vi "FGGA TCP Packet_v3.3.vi"(0 "ID":string, 5 "Version":string, 7 "TCP Packet In":string, 9 "utc_time":u32, 12 "Data Array":string[](array[string])) -> (8 "TCP Binary Packet":string)   [LabVIEW 2014]
panel:
  out "array":string[](array[string])
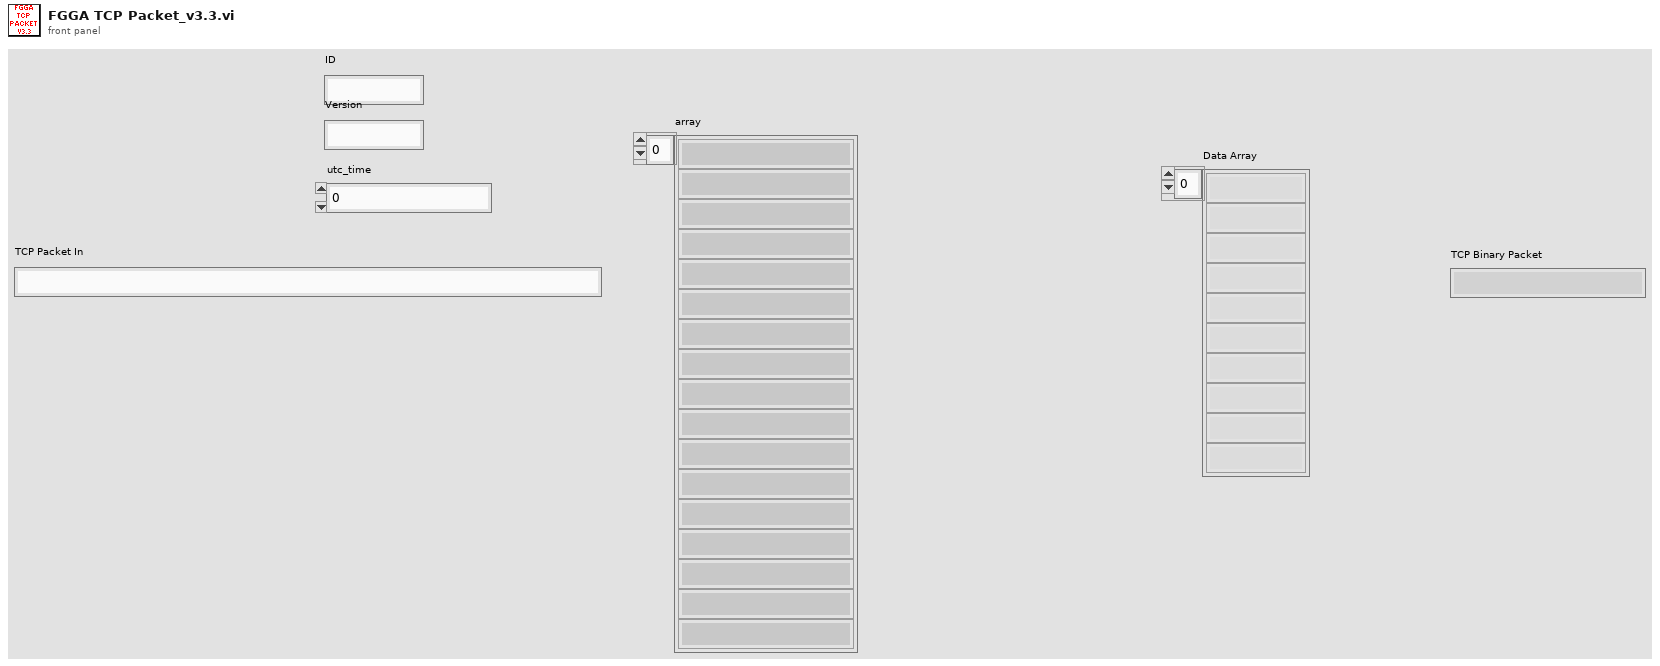
[diagram p1: front panel]
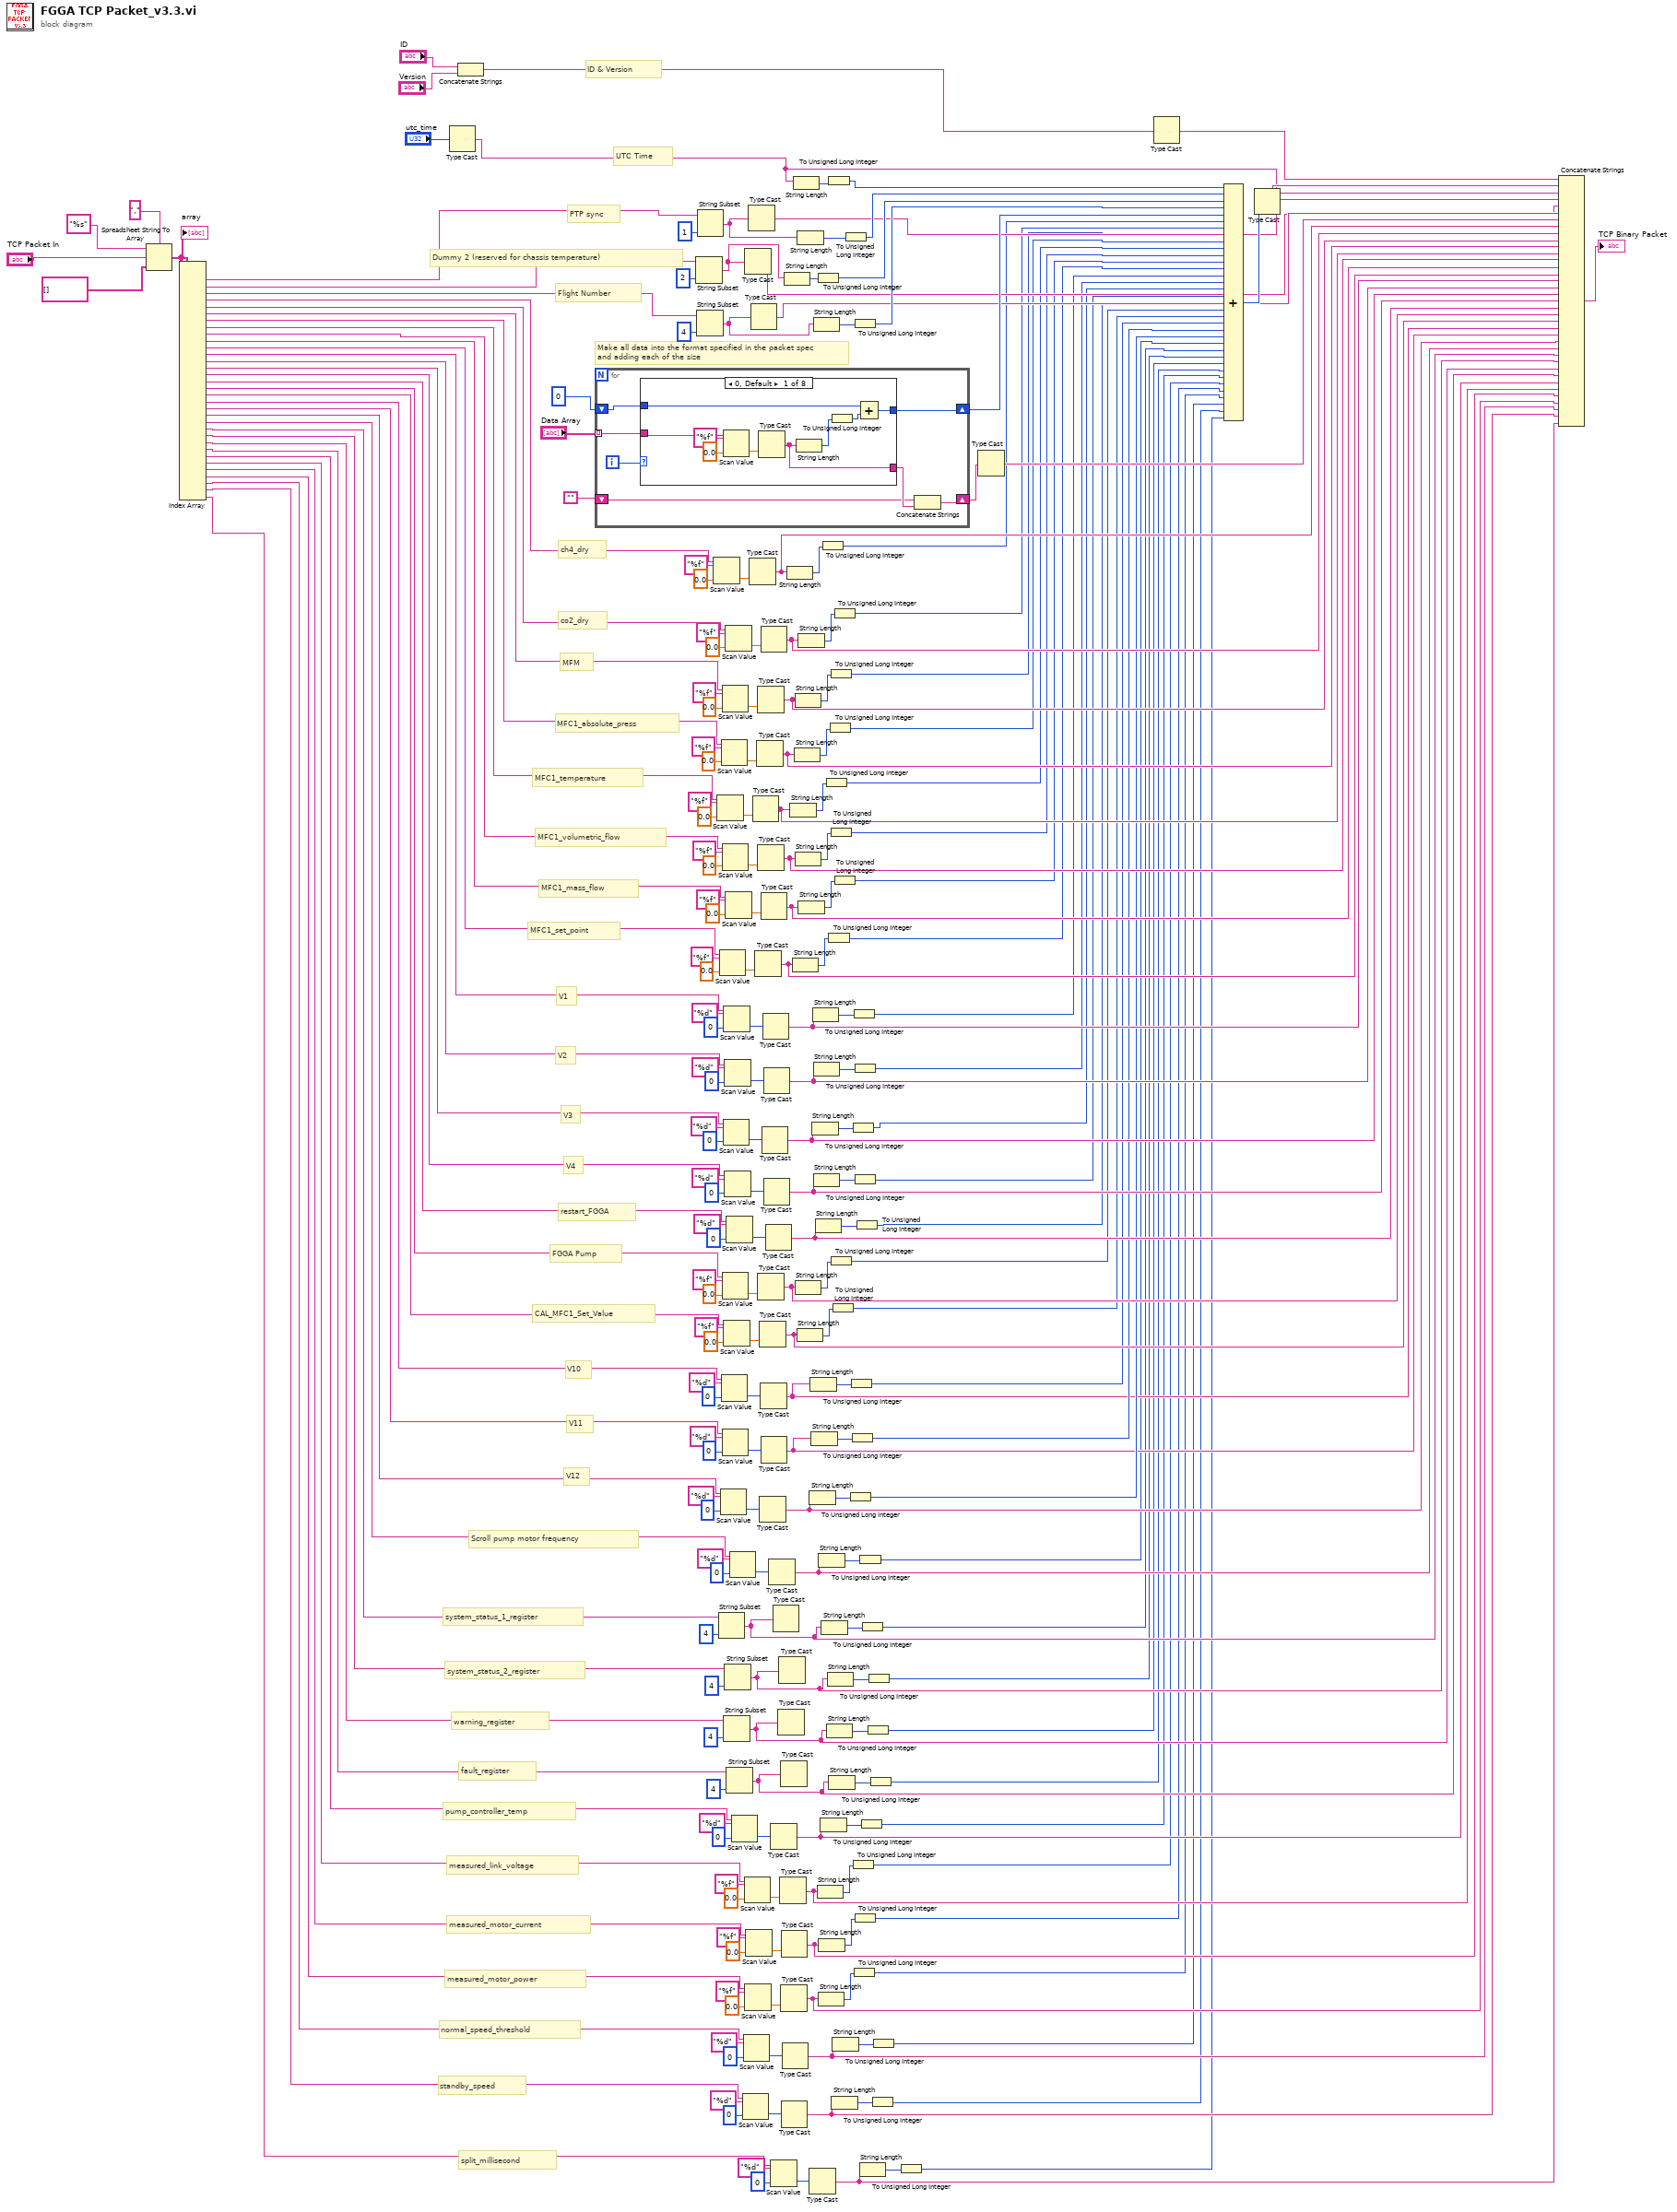
[diagram p0: block diagram]
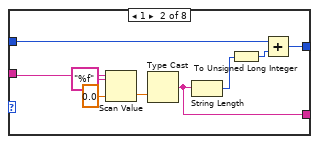
[diagram p2: hidden frame]
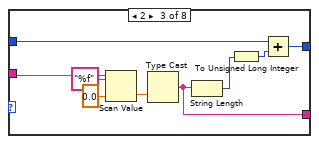
[diagram p3: hidden frame]
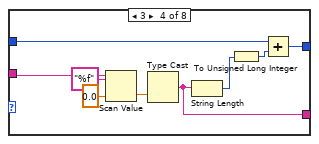
[diagram p4: hidden frame]
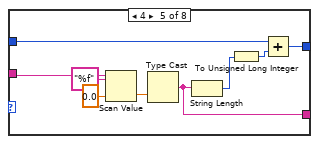
[diagram p5: hidden frame]
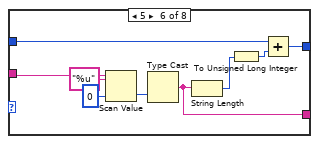
[diagram p6: hidden frame]
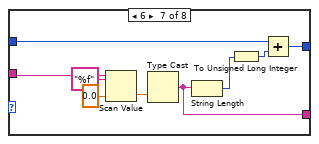
[diagram p7: hidden frame]
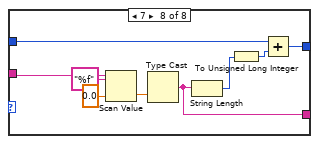
[diagram p8: hidden frame]
diagram:
  # "split_millisecond"
  # "standby_speed"
  # "normal_speed_threshold"
  # "measured_motor_power"
  # "measured_motor_current"
  # "measured_link_voltage"
  # "pump_controller_temp"
  # "fault_register"
  # "warning_register"
  # "system_status_2_register"
  # "system_status_1_register"
  # "Scroll pump motor frequency"
  # "V12"
  # "V11"
  # "V10"
  # "PTP sync"
  # "CAL_MFC1_Set_Value"
  # "FGGA Pump"
  # "restart_FGGA"
  # "V4"
  # "V3"
  # "V2"
  # "V1"
  # "MFC1_set_point"
  # "MFC1_mass_flow"
  # "MFC1_volumetric_flow"
  # "MFC1_temperature"
  # "MFC1_absolute_press"
  # "MFM"
  # "co2_dry"
  # "ch4_dry"
  # "Flight Number"
  # "Dummy 2 (reserved for chassis temperature)"
  # "UTC Time"
  # "ID & Version"
  # "Make all data into the format specified in the packet spec\nand adding each of the size"
  n1 = Spreadsheet String To Array(delimiter (Tab)=",", format string="%s", spreadsheet string="TCP Packet In", array type (2D Dbl)=string[] []) -> (array=w199:string[])
  "array" <- w199
  n2 = Index Array(array=w199) -> (element #1=w198:string, element #2=w197:string, element #3=w196:string, element #4=w195:string, element #5=w194:string, element #6=w169:string, element #7=w166:string, element #8=w163:string, element #9=w160:string, element #10=w157:string, element #11=w154:string, element #12=w147:string, element #13=w140:string, element #14=w117:string, element #15=w114:string, element #16=w111:string, element #17=w108:string, element #18=w105:string, element #19=w85:string, element #20=w84:string, element #21=w83:string, element #22=w40:string, element #23=w39:string, element #24=w38:string, element #25=w37:string, element #26=w36:string, element #27=w35:string, element #28=w34:string, element #29=w33:string, element #30=w32:string, element #31=w31:string, element #32=w30:string, element #33=w3:string)  [unwired: 33 in]
  n3 = Type Cast(x="utc_time") -> (*(type *) &x=w98:string)  [unwired: 1 in]
  n4 = Concatenate Strings("ID", "Version") -> (w100:string)
  n5 = for {
    tunnel: "Data Array" -> [w248] mode=indexing
    shift-right: [w246] -> w230
    shift-left: u32 0 -> [w247]
    shift-right: [w245] -> w219
    shift-left: "" -> [w243]
    i -> [w249]
    n6 = case shown="0, Default" w249 {
      tunnel: w248 -> [w256 w265 w274 w283 w292 w301 w310 w319]
      tunnel: w247 -> [w254 w263 w272 w281 w290 w299 w308 w317]
      tunnel: [w251 w260 w269 w278 w287 w296 w305 w314] -> w246
      tunnel: [w250 w259 w268 w277 w286 w295 w304 w313] -> w244
      frame 0, Default {
        n7 = Scan Value(string=w256, format string="%f", default (0 dbl)=sgl 0.0 ("default (0 I32)")) -> (value=w258:sgl)  [unwired: 1 out]
        n8 = Type Cast(x=w258) -> (*(type *) &x=w250:string)  [unwired: 1 in]
        n9 = String Length(string=w250) -> (length=w253:i32)
        n10 = To Unsigned Long Integer(number=w253) -> (unsigned 32bit integer=w252:u32)
        n11 = Add(x=w254, y=w252) -> (x+y=w251:u32)
      }
      frame 1 {
        n12 = Scan Value(string=w265, format string="%f", default (0 dbl)=sgl 0.0 ("default (0 I32)")) -> (value=w267:sgl)  [unwired: 1 out]
        n13 = Type Cast(x=w267) -> (*(type *) &x=w259:string)  [unwired: 1 in]
        n14 = String Length(string=w259) -> (length=w262:i32)
        n15 = To Unsigned Long Integer(number=w262) -> (unsigned 32bit integer=w261:u32)
        n16 = Add(x=w263, y=w261) -> (x+y=w260:u32)
      }
      frame 2 {
        n17 = Scan Value(string=w274, format string="%f", default (0 dbl)=sgl 0.0 ("default (0 I32)")) -> (value=w276:sgl)  [unwired: 1 out]
        n18 = Type Cast(x=w276) -> (*(type *) &x=w268:string)  [unwired: 1 in]
        n19 = String Length(string=w268) -> (length=w271:i32)
        n20 = To Unsigned Long Integer(number=w271) -> (unsigned 32bit integer=w270:u32)
        n21 = Add(x=w272, y=w270) -> (x+y=w269:u32)
      }
      frame 3 {
        n22 = Scan Value(string=w283, format string="%f", default (0 dbl)=sgl 0.0 ("default (0 I32)")) -> (value=w285:sgl)  [unwired: 1 out]
        n23 = Type Cast(x=w285) -> (*(type *) &x=w277:string)  [unwired: 1 in]
        n24 = String Length(string=w277) -> (length=w280:i32)
        n25 = To Unsigned Long Integer(number=w280) -> (unsigned 32bit integer=w279:u32)
        n26 = Add(x=w281, y=w279) -> (x+y=w278:u32)
      }
      frame 4 {
        n27 = Scan Value(string=w292, format string="%f", default (0 dbl)=sgl 0.0 ("default (0 I32)")) -> (value=w294:sgl)  [unwired: 1 out]
        n28 = Type Cast(x=w294) -> (*(type *) &x=w286:string)  [unwired: 1 in]
        n29 = String Length(string=w286) -> (length=w289:i32)
        n30 = To Unsigned Long Integer(number=w289) -> (unsigned 32bit integer=w288:u32)
        n31 = Add(x=w290, y=w288) -> (x+y=w287:u32)
      }
      frame 5 {
        n32 = Scan Value(string=w301, format string="%u", default (0 dbl)=u16 0 ("default (0 I32)")) -> (value=w303:u16)  [unwired: 1 out]
        n33 = Type Cast(x=w303) -> (*(type *) &x=w295:string)  [unwired: 1 in]
        n34 = String Length(string=w295) -> (length=w298:i32)
        n35 = To Unsigned Long Integer(number=w298) -> (unsigned 32bit integer=w297:u32)
        n36 = Add(x=w299, y=w297) -> (x+y=w296:u32)
      }
      frame 6 {
        n37 = Scan Value(string=w310, format string="%f", default (0 dbl)=sgl 0.0 ("default (0 I32)")) -> (value=w312:sgl)  [unwired: 1 out]
        n38 = Type Cast(x=w312) -> (*(type *) &x=w304:string)  [unwired: 1 in]
        n39 = String Length(string=w304) -> (length=w307:i32)
        n40 = To Unsigned Long Integer(number=w307) -> (unsigned 32bit integer=w306:u32)
        n41 = Add(x=w308, y=w306) -> (x+y=w305:u32)
      }
      frame 7 {
        n42 = Scan Value(string=w319, format string="%f", default (0 dbl)=sgl 0.0 ("default (0 I32)")) -> (value=w321:sgl)  [unwired: 1 out]
        n43 = Type Cast(x=w321) -> (*(type *) &x=w313:string)  [unwired: 1 in]
        n44 = String Length(string=w313) -> (length=w316:i32)
        n45 = To Unsigned Long Integer(number=w316) -> (unsigned 32bit integer=w315:u32)
        n46 = Add(x=w317, y=w315) -> (x+y=w314:u32)
      }
    }
    n47 = Concatenate Strings(w243, w244) -> (w245:string)
  }
  n48 = String Subset(string=w197, length (rest)=2 ("length (rest)")) -> (substring=w217:string)  [unwired: 1 in]
  n49 = String Subset(string=w196, length (rest)=4 ("length (rest)")) -> (substring=w223:string)  [unwired: 1 in]
  n50 = String Subset(string=w198, length (rest)=1 ("length (rest)")) -> (substring=w226:string)  [unwired: 1 in]
  n51 = Scan Value(string=w195, format string="%f", default (0 dbl)=sgl 0.0 ("default (0 I32)")) -> (value=w215:sgl)  [unwired: 1 out]
  n52 = Scan Value(string=w163, format string="%f", default (0 dbl)=sgl 0.0 ("default (0 I32)")) -> (value=w185:sgl)  [unwired: 1 out]
  n53 = String Subset(string=w39, length (rest)=4 ("length (rest)")) -> (substring=w26:string)  [unwired: 1 in]
  n54 = Scan Value(string=w154, format string="%f", default (0 dbl)=sgl 0.0 ("default (0 I32)")) -> (value=w173:sgl)  [unwired: 1 out]
  n55 = Scan Value(string=w83, format string="%d", default (0 dbl)=u16 0 ("default (0 I32)")) -> (value=w86:u16)  [unwired: 1 out]
  n56 = Scan Value(string=w166, format string="%f", default (0 dbl)=sgl 0.0 ("default (0 I32)")) -> (value=w189:sgl)  [unwired: 1 out]
  n57 = Scan Value(string=w85, format string="%d", default (0 dbl)=u16 0 ("default (0 I32)")) -> (value=w94:u16)  [unwired: 1 out]
  n58 = Scan Value(string=w169, format string="%f", default (0 dbl)=sgl 0.0 ("default (0 I32)")) -> (value=w193:sgl)  [unwired: 1 out]
  n59 = Scan Value(string=w160, format string="%f", default (0 dbl)=sgl 0.0 ("default (0 I32)")) -> (value=w181:sgl)  [unwired: 1 out]
  n60 = Scan Value(string=w108, format string="%f", default (0 dbl)=sgl 0.0 ("default (0 I32)")) -> (value=w125:sgl)  [unwired: 1 out]
  n61 = Scan Value(string=w84, format string="%d", default (0 dbl)=u16 0 ("default (0 I32)")) -> (value=w90:u16)  [unwired: 1 out]
  n62 = Scan Value(string=w117, format string="%d", default (0 dbl)=u16 0 ("default (0 I32)")) -> (value=w134:u16)  [unwired: 1 out]
  n63 = Scan Value(string=w147, format string="%d", default (0 dbl)=u16 0 ("default (0 I32)")) -> (value=w148:u16)  [unwired: 1 out]
  n64 = Scan Value(string=w105, format string="%f", default (0 dbl)=sgl 0.0 ("default (0 I32)")) -> (value=w121:sgl)  [unwired: 1 out]
  n65 = String Subset(string=w37, length (rest)=4 ("length (rest)")) -> (substring=w22:string)  [unwired: 1 in]
  n66 = Scan Value(string=w140, format string="%d", default (0 dbl)=u16 0 ("default (0 I32)")) -> (value=w141:u16)  [unwired: 1 out]
  n67 = Scan Value(string=w114, format string="%d", default (0 dbl)=u16 0 ("default (0 I32)")) -> (value=w130:u16)  [unwired: 1 out]
  n68 = String Subset(string=w38, length (rest)=4 ("length (rest)")) -> (substring=w24:string)  [unwired: 1 in]
  n69 = Scan Value(string=w194, format string="%f", default (0 dbl)=sgl 0.0 ("default (0 I32)")) -> (value=w209:sgl)  [unwired: 1 out]
  n70 = Scan Value(string=w157, format string="%f", default (0 dbl)=sgl 0.0 ("default (0 I32)")) -> (value=w177:sgl)  [unwired: 1 out]
  n71 = Scan Value(string=w111, format string="%d", default (0 dbl)=u16 0 ("default (0 I32)")) -> (value=w126:u16)  [unwired: 1 out]
  n72 = String Subset(string=w36, length (rest)=4 ("length (rest)")) -> (substring=w20:string)  [unwired: 1 in]
  n73 = Scan Value(string=w40, format string="%d", default (0 dbl)=u16 0 ("default (0 I32)")) -> (value=w73:u16)  [unwired: 1 out]
  n74 = Scan Value(string=w35, format string="%d", default (0 dbl)=u16 0 ("default (0 I32)")) -> (value=w61:u16)  [unwired: 1 out]
  n75 = Scan Value(string=w30, format string="%d", default (0 dbl)=u16 0 ("default (0 I32)")) -> (value=w41:u16)  [unwired: 1 out]
  n76 = Scan Value(string=w31, format string="%d", default (0 dbl)=u16 0 ("default (0 I32)")) -> (value=w45:u16)  [unwired: 1 out]
  n77 = Scan Value(string=w34, format string="%f", default (0 dbl)=sgl 0.0 ("default (0 I32)")) -> (value=w60:sgl)  [unwired: 1 out]
  n78 = Type Cast(x=w217) -> (*(type *) &x=w216:string)  [unwired: 1 in]
  n79 = Scan Value(string=w32, format string="%f", default (0 dbl)=sgl 0.0 ("default (0 I32)")) -> (value=w52:sgl)  [unwired: 1 out]
  n80 = Scan Value(string=w33, format string="%f", default (0 dbl)=sgl 0.0 ("default (0 I32)")) -> (value=w56:sgl)  [unwired: 1 out]
  n81 = Type Cast(x=w226) -> (*(type *) &x=w225:string)  [unwired: 1 in]
  n82 = Type Cast(x=w215) -> (*(type *) &x=w211:string)  [unwired: 1 in]
  n83 = Type Cast(x=w223) -> (*(type *) &x=w224:string)  [unwired: 1 in]
  n84 = Type Cast(x=w185) -> (*(type *) &x=w161:string)  [unwired: 1 in]
  n85 = Type Cast(x=w173) -> (*(type *) &x=w152:string)  [unwired: 1 in]
  n86 = Type Cast(x=w189) -> (*(type *) &x=w164:string)  [unwired: 1 in]
  n87 = Type Cast(x=w193) -> (*(type *) &x=w167:string)  [unwired: 1 in]
  n88 = Type Cast(x=w181) -> (*(type *) &x=w158:string)  [unwired: 1 in]
  n89 = Type Cast(x=w125) -> (*(type *) &x=w106:string)  [unwired: 1 in]
  n90 = Type Cast(x=w121) -> (*(type *) &x=w103:string)  [unwired: 1 in]
  n91 = Type Cast(x=w86) -> (*(type *) &x=w77:string)  [unwired: 1 in]
  n92 = Type Cast(x=w94) -> (*(type *) &x=w79:string)  [unwired: 1 in]
  n93 = Type Cast(x=w209) -> (*(type *) &x=w204:string)  [unwired: 1 in]
  n94 = Type Cast(x=w177) -> (*(type *) &x=w155:string)  [unwired: 1 in]
  n95 = Type Cast(x=w90) -> (*(type *) &x=w78:string)  [unwired: 1 in]
  n96 = Type Cast(x=w134) -> (*(type *) &x=w115:string)  [unwired: 1 in]
  n97 = Type Cast(x=w148) -> (*(type *) &x=w145:string)  [unwired: 1 in]
  n98 = Type Cast(x=w141) -> (*(type *) &x=w138:string)  [unwired: 1 in]
  n99 = Type Cast(x=w130) -> (*(type *) &x=w112:string)  [unwired: 1 in]
  n100 = Type Cast(x=w126) -> (*(type *) &x=w109:string)  [unwired: 1 in]
  n101 = Type Cast(x=w73) -> (*(type *) &x=w28:string)  [unwired: 1 in]
  n102 = Type Cast(x=w61) -> (*(type *) &x=w18:string)  [unwired: 1 in]
  n103 = Scan Value(string=w3, format string="%d", default (0 dbl)=u16 0 ("default (0 I32)")) -> (value=w4:u16)  [unwired: 1 out]
  n104 = Type Cast(x=w26) -> ()  [unwired: 1 in, 1 out]
  n105 = Type Cast(x=w22) -> ()  [unwired: 1 in, 1 out]
  n106 = Type Cast(x=w24) -> ()  [unwired: 1 in, 1 out]
  n107 = Type Cast(x=w60) -> (*(type *) &x=w16:string)  [unwired: 1 in]
  n108 = Type Cast(x=w20) -> ()  [unwired: 1 in, 1 out]
  n109 = Type Cast(x=w52) -> (*(type *) &x=w12:string)  [unwired: 1 in]
  n110 = Type Cast(x=w56) -> (*(type *) &x=w14:string)  [unwired: 1 in]
  n111 = Type Cast(x=w41) -> (*(type *) &x=w8:string)  [unwired: 1 in]
  n112 = Type Cast(x=w45) -> (*(type *) &x=w10:string)  [unwired: 1 in]
  n113 = String Length(string=w217) -> (length=w237:i32)
  n114 = String Length(string=w211) -> (length=w212:i32)
  n115 = String Length(string=w161) -> (length=w182:i32)
  n116 = String Length(string=w152) -> (length=w170:i32)
  n117 = String Length(string=w98) -> (length=w242:i32)
  n118 = String Length(string=w164) -> (length=w186:i32)
  n119 = String Length(string=w167) -> (length=w190:i32)
  n120 = String Length(string=w158) -> (length=w178:i32)
  n121 = String Length(string=w106) -> (length=w122:i32)
  n122 = String Length(string=w103) -> (length=w118:i32)
  n123 = String Length(string=w226) -> (length=w239:i32)
  n124 = String Length(string=w204) -> (length=w206:i32)
  n125 = String Length(string=w155) -> (length=w174:i32)
  n126 = String Length(string=w77) -> (length=w89:i32)
  n127 = Type Cast(x=w4) -> (*(type *) &x=w1:string)  [unwired: 1 in]
  n128 = String Length(string=w79) -> (length=w97:i32)
  n129 = String Length(string=w78) -> (length=w93:i32)
  n130 = String Length(string=w115) -> (length=w137:i32)
  n131 = String Length(string=w145) -> (length=w151:i32)
  n132 = String Length(string=w223) -> (length=w234:i32)
  n133 = String Length(string=w138) -> (length=w144:i32)
  n134 = String Length(string=w112) -> (length=w133:i32)
  n135 = To Unsigned Long Integer(number=w237) -> (unsigned 32bit integer=w236:u32)
  n136 = String Length(string=w109) -> (length=w129:i32)
  n137 = String Length(string=w16) -> (length=w57:i32)
  n138 = String Length(string=w12) -> (length=w49:i32)
  n139 = String Length(string=w28) -> (length=w76:i32)
  n140 = String Length(string=w14) -> (length=w53:i32)
  n141 = To Unsigned Long Integer(number=w212) -> (unsigned 32bit integer=w210:u32)
  n142 = String Length(string=w18) -> (length=w64:i32)
  n143 = String Length(string=w26) -> (length=w71:i32)
  n144 = To Unsigned Long Integer(number=w182) -> (unsigned 32bit integer=w162:u32)
  n145 = To Unsigned Long Integer(number=w242) -> (unsigned 32bit integer=w241:u32)
  n146 = To Unsigned Long Integer(number=w170) -> (unsigned 32bit integer=w153:u32)
  n147 = String Length(string=w22) -> (length=w67:i32)
  n148 = To Unsigned Long Integer(number=w186) -> (unsigned 32bit integer=w165:u32)
  n149 = String Length(string=w24) -> (length=w69:i32)
  n150 = To Unsigned Long Integer(number=w190) -> (unsigned 32bit integer=w168:u32)
  n151 = To Unsigned Long Integer(number=w178) -> (unsigned 32bit integer=w159:u32)
  n152 = To Unsigned Long Integer(number=w122) -> (unsigned 32bit integer=w107:u32)
  n153 = String Length(string=w20) -> (length=w65:i32)
  n154 = To Unsigned Long Integer(number=w118) -> (unsigned 32bit integer=w104:u32)
  n155 = To Unsigned Long Integer(number=w206) -> (unsigned 32bit integer=w205:u32)
  n156 = To Unsigned Long Integer(number=w174) -> (unsigned 32bit integer=w156:u32)
  n157 = String Length(string=w8) -> (length=w44:i32)
  n158 = String Length(string=w10) -> (length=w48:i32)
  n159 = To Unsigned Long Integer(number=w239) -> (unsigned 32bit integer=w238:u32)
  n160 = To Unsigned Long Integer(number=w89) -> (unsigned 32bit integer=w80:u32)
  n161 = To Unsigned Long Integer(number=w97) -> (unsigned 32bit integer=w82:u32)
  n162 = To Unsigned Long Integer(number=w93) -> (unsigned 32bit integer=w81:u32)
  n163 = To Unsigned Long Integer(number=w137) -> (unsigned 32bit integer=w116:u32)
  n164 = To Unsigned Long Integer(number=w57) -> (unsigned 32bit integer=w17:u32)
  n165 = To Unsigned Long Integer(number=w151) -> (unsigned 32bit integer=w146:u32)
  n166 = To Unsigned Long Integer(number=w49) -> (unsigned 32bit integer=w13:u32)
  n167 = To Unsigned Long Integer(number=w234) -> (unsigned 32bit integer=w233:u32)
  n168 = To Unsigned Long Integer(number=w144) -> (unsigned 32bit integer=w139:u32)
  n169 = To Unsigned Long Integer(number=w133) -> (unsigned 32bit integer=w113:u32)
  n170 = To Unsigned Long Integer(number=w53) -> (unsigned 32bit integer=w15:u32)
  n171 = To Unsigned Long Integer(number=w129) -> (unsigned 32bit integer=w110:u32)
  n172 = To Unsigned Long Integer(number=w76) -> (unsigned 32bit integer=w29:u32)
  n173 = To Unsigned Long Integer(number=w64) -> (unsigned 32bit integer=w19:u32)
  n174 = To Unsigned Long Integer(number=w71) -> (unsigned 32bit integer=w27:u32)
  n175 = String Length(string=w1) -> (length=w7:i32)
  n176 = To Unsigned Long Integer(number=w67) -> (unsigned 32bit integer=w23:u32)
  n177 = To Unsigned Long Integer(number=w69) -> (unsigned 32bit integer=w25:u32)
  n178 = To Unsigned Long Integer(number=w65) -> (unsigned 32bit integer=w21:u32)
  n179 = To Unsigned Long Integer(number=w44) -> (unsigned 32bit integer=w9:u32)
  n180 = To Unsigned Long Integer(number=w48) -> (unsigned 32bit integer=w11:u32)
  n181 = To Unsigned Long Integer(number=w7) -> (unsigned 32bit integer=w2:u32)
  n182 = Type Cast(x=w219) -> (*(type *) &x=w222:string)  [unwired: 1 in]
  n183 = Type Cast(x=w100) -> (*(type *) &x=w229:string)  [unwired: 1 in]
  n184 = Compound Arithmetic op=ADD(w241, w238, w236, w233, w230, w210, w205, w168, w165, w162, w159, w156, w153, w146, w139, w116, w113, w110, w107, w104, w82, w81, w80, w29, w27, w25, w23, w21, w19, w17, w15, w13, w11, w9, w2) -> (w228:u32)
  n185 = Type Cast(x=w228) -> (*(type *) &x=w227:string)  [unwired: 1 in]
  n186 = Concatenate Strings(w229, w227, w98, w225, w216, w224, w222, w211, w204, w167, w164, w161, w158, w155, w152, w145, w138, w115, w112, w109, w106, w103, w79, w78, w77, w28, w26, w24, w22, w20, w18, w16, w14, w12, w10, w8, w1) -> (→"TCP Binary Packet":string)
